vi "2_Cross_Correlation.vi"(8 "error in (no error)":errorcluster) -> (0 "error out":errorcluster)   [LabVIEW 2014]
uses:
  SwabianInstruments.TimeTagger
panel:
  out "Cross correlation":cluster{dbl[], "getData":i32[]}(graph)
  # "cross correlation between channels 1 and 2\nbinwidth=1000 ps, n_bins=3000, thus we sample 3000 ns\nwe should see the correlation delta peaks at a bit more than 1000 ns distance"
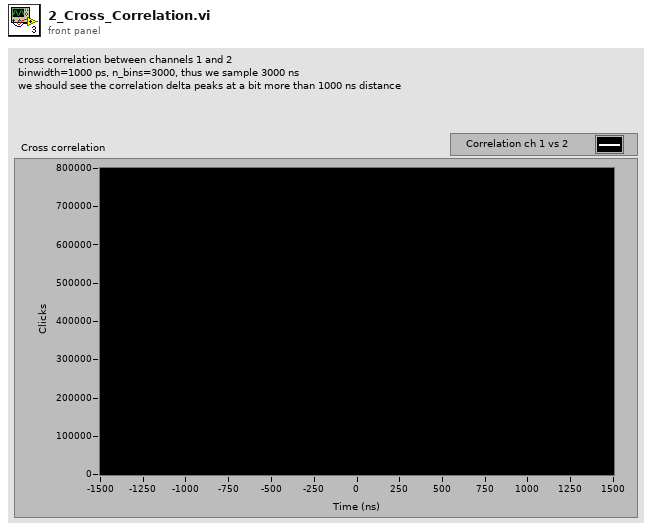
[diagram p1: front panel]
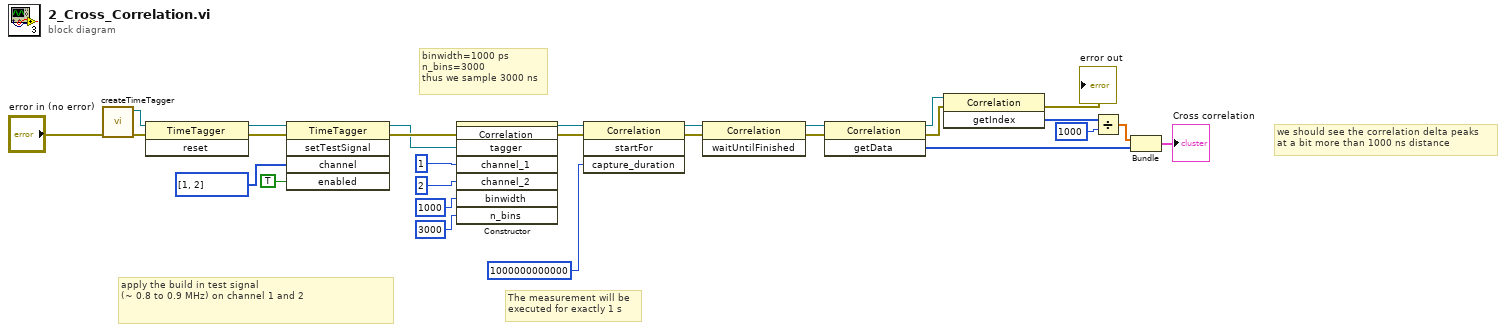
[diagram p0: block diagram]
diagram:
  # "The measurement will be\nexecuted for exactly 1 s"
  # "we should see the correlation delta peaks \nat a bit more than 1000 ns distance"
  # "apply the build in test signal\n(~ 0.8 to 0.9 MHz) on channel 1 and 2"
  # "binwidth=1000 ps\nn_bins=3000\nthus we sample 3000 ns"
  n1 = call "createTimeTagger.vi"("error in (no error)"="error in (no error)") -> ("error out"=w14:errorcluster, "TimeTagger ref out"=w15:refnum<k24>)  [unwired: 9 in]
  n2 = invoke class="TimeTagger" method="reset"(reference=w15, error in=w14) -> (reference out=w24:refnum<k24>, error out=w23:errorcluster)  [unwired: 1 in, 1 out]
  n3 = invoke class="TimeTagger" method="setTestSignal"(reference=w24, error in=w23, "channel"=i32[] [1, 2], "enabled"=TRUE) -> (reference out=w13:refnum<k24>, error out=w20:errorcluster)  [unwired: 1 in, 3 out]
  n4 = constructor class="Correlation"(error in=w20, "tagger"=w13, "channel_1"=1, "channel_2"=2, "binwidth"=i64 1000, "n_bins"=3000) -> (reference out=w9:refnum<k24>, error out=w7:errorcluster)  [unwired: 2 in, 6 out]
  n5 = invoke class="Correlation" method="startFor"(reference=w9, error in=w7, "capture_duration"=i64 1000000000000) -> (reference out=w4:refnum<k24>, error out=w3:errorcluster)  [unwired: 1 in, 2 out]
  n6 = invoke class="Correlation" method="waitUntilFinished"(reference=w4, error in=w3) -> (reference out=w6:refnum<k24>, error out=w5:errorcluster)  [unwired: 1 in, 1 out]
  n7 = invoke class="Correlation" method="getData"(reference=w6, error in=w5) -> (reference out=w28:refnum<k24>, error out=w27:errorcluster, "getData"=w10:i32[])  [unwired: 1 in]
  n8 = invoke class="Correlation" method="getIndex"(reference=w28, error in=w27) -> (error out=→"error out":errorcluster, "getIndex"=w25:i64[])  [unwired: 1 in, 1 out]
  n9 = Divide(x=w25, y=i64 1000) -> (x/y=w11:dbl[])
  n10 = Bundle(w11, "getData"=w10) -> (→"Cross correlation":cluster{dbl[], "getData":i32[]})  [unwired: 1 in]
